vi "Check Library Owner.vi"(8 "Error in":errorcluster caption="Error in (no error)", 10 "Library":refnum<vi>, 11 "VIDoc Parser In":refnum<class "VIDoc Parser.lvclass">) -> (0 "Error out":errorcluster, 3 "VIDoc Parser Out":refnum<class "VIDoc Parser.lvclass">)   [LabVIEW 2023, in "VIDoc Parsing.lvlib" / "VIDoc Parser.lvclass"]
uses:
  VIDoc Parser.lvclass
  VIDoc Parser.lvclass/VIDoc Parser.ctl
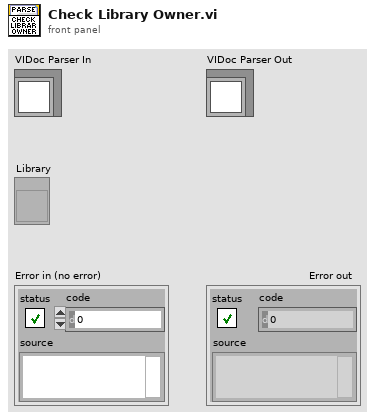
[diagram p1: front panel]
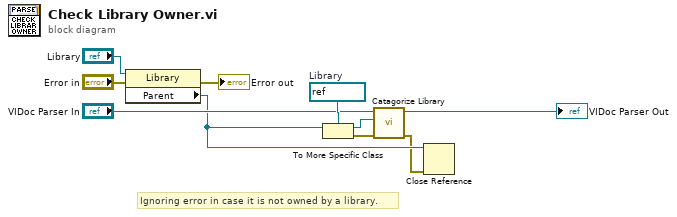
[diagram p0: block diagram]
diagram:
  w10 = refnum<vi> refnum  # Library
  # "Ignoring error in case it is not owned by a library."
  n1 = property class="Library"(reference="Library", error in="Error in") -> (error out=→"Error out":errorcluster, "Parent"=w2:refnum<vi>)  [unwired: 1 out]
  n2 = To More Specific Class(target class=w10, reference=w2) -> (specific class reference=w9:refnum<vi>, error out=w8:errorcluster)  [unwired: 1 in]
  n3 = call "Catagorize Library.vi"("error in (no error)"=w8, "Library"=w9, "VIDoc Parser In"="VIDoc Parser In") -> ("error out"=w1:errorcluster, "VIDoc Parser Out"=→"VIDoc Parser Out":refnum<class "VIDoc Parser.lvclass">)  [unwired: 6 in, 1 out]
  n4 = Close Reference(reference=w2, error in (no error)=w1) -> ()  [unwired: 1 out]
